vi "set waittime.vi"(8 "error in":errorcluster, 11 "Lock-In Amplifier":refnum<class "Lock-In Amplifier.lvclass">) -> (0 "error out":errorcluster, 2 "Wait time":u32, 3 "Lock-In Amplifier":refnum<class "Lock-In Amplifier.lvclass">)   [LabVIEW 2020, in "Lock-In Amplifier.lvclass"]
uses:
  Lock-In Amplifier.lvclass
  Lock-In Amplifier.lvclass/Lock-In Amplifier.ctl
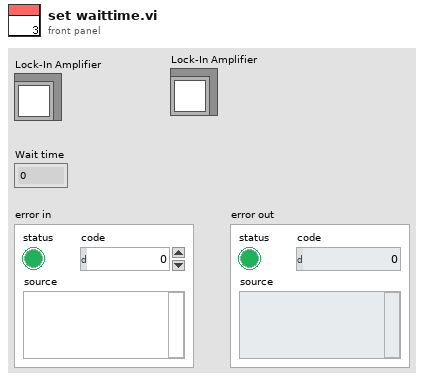
[diagram p1: front panel]
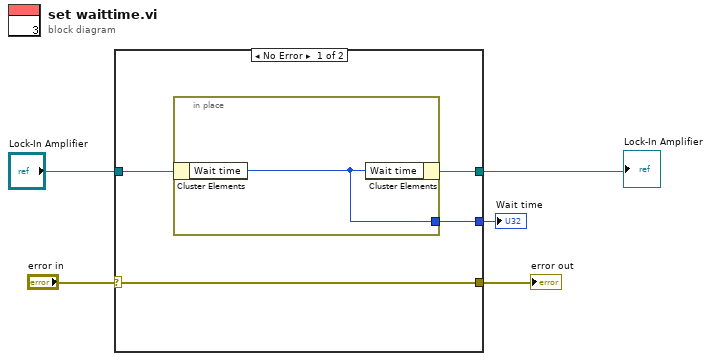
[diagram p0: block diagram]
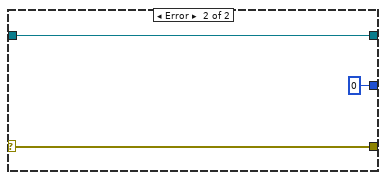
[diagram p2: hidden frame]
diagram:
  n1 = case shown="No Error" "error in" {
    selector: "error in" -> [w7 w12]
    tunnel: "Lock-In Amplifier" -> [w9 w13]
    tunnel: [w8 w13] -> w4
    tunnel: [w7 w12] -> w2
    tunnel: [w6 u32 0 ("Wait time")] -> w1
    frame No Error {
      n2 = in-place {
        in-place-border: [w10] -> w6
        n3 = in-place-cluster #1(w9) -> ("Wait time"=w10:u32)
        n4 = in-place-cluster #1("Wait time"=w10) -> (w8:refnum<class "Lock-In Amplifier.lvclass">)
      }
    }
    frame Error {
    }
  }
  "Lock-In Amplifier" <- w4
  "error out" <- w2
  "Wait time" <- w1
